vi "Final Project GUI SIM VERSION .vi"() -> ()   [LabVIEW 2021]
uses:
  <vilib>/picture/picture.llb/Draw True-Color Pixmap.vi
  <vilib>/addons/control/pid/NI_PID_pid.lvlib
  <vilib>/addons/control/pid/pid.llb/PID (DBL).vi
panel:
  out "Rear Left Actuator":string
  out "Front Left Actuator":string
  out "Rear Right Actuator":string
  out "Front Right Actuator":string
  in  "Back Button":bool
  in  "Right Button":bool
  in  "Front Button":bool
  in  "Left Button":bool
  in  "PID gains":T1={"proportional gain (Kc)"=20.0, "integral time (Ti, min)"=0.008, "derivative time (Td, min)"=0.001} {"derivative time (Td, min)" format="%.3f"; "integral time (Ti, min)" format="%.3f"; "proportional gain (Kc)" format="%.3f"}
  out "Side View":picture
  out "24-bit pixmap":u32[][](array[numeric]) format="%x"
  out "Front View":picture
  in  "Stop":bool
  # "DISTURBANCE CREATOR\n(Press a button to introduce a bump on that specific side)"
  # "CAR"
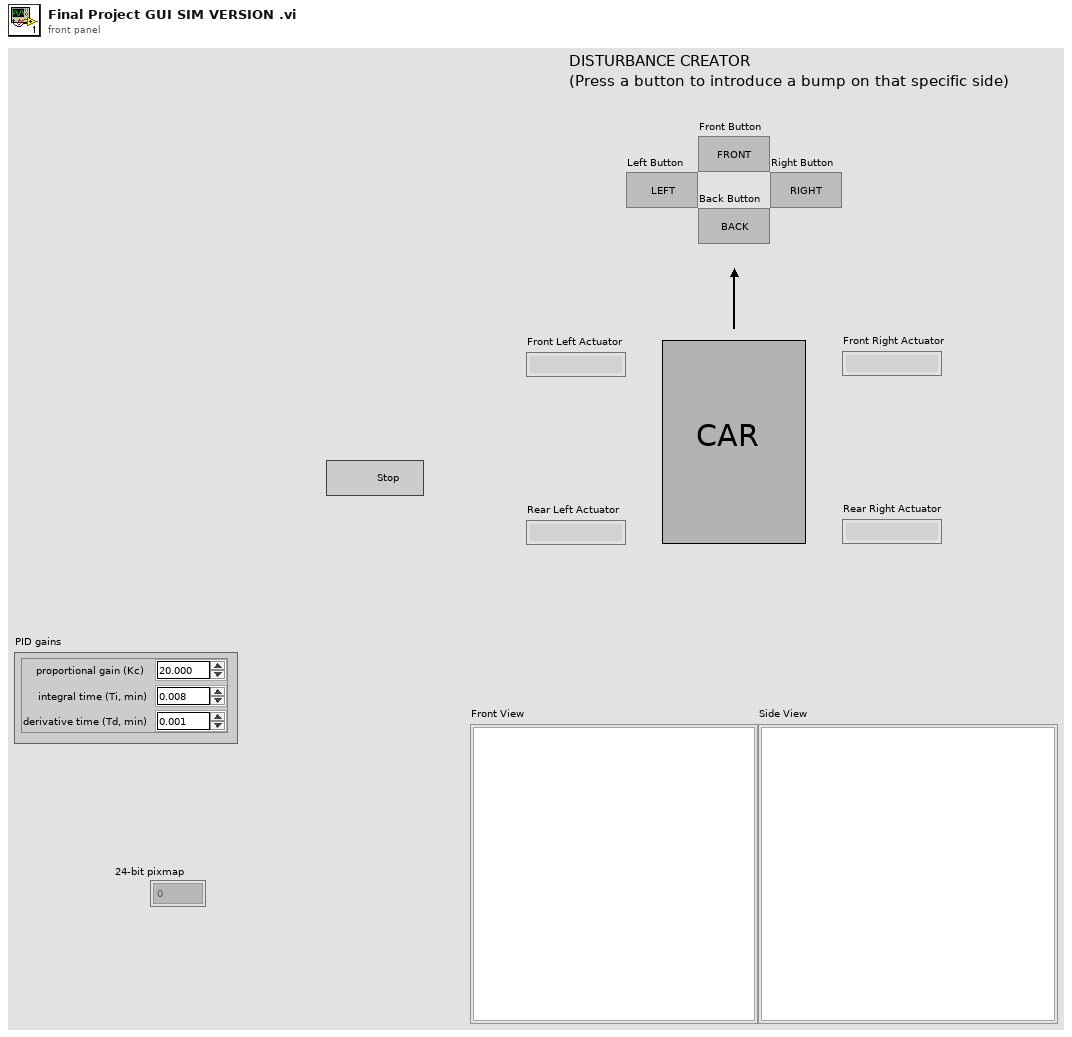
[diagram p1: front panel]
types:
  T1 = cluster{"proportional gain (Kc)":dbl, "integral time (Ti, min)":dbl, "derivative time (Td, min)":dbl}
  T2 = typedef "imagedata.ctl" = cluster{"image type":i32, "image depth":i32, "image":u8[], "mask":u8[], "colors":u32[], "Rectangle":cluster{"left":i16, "top":i16, "right":i16, "bottom":i16}}
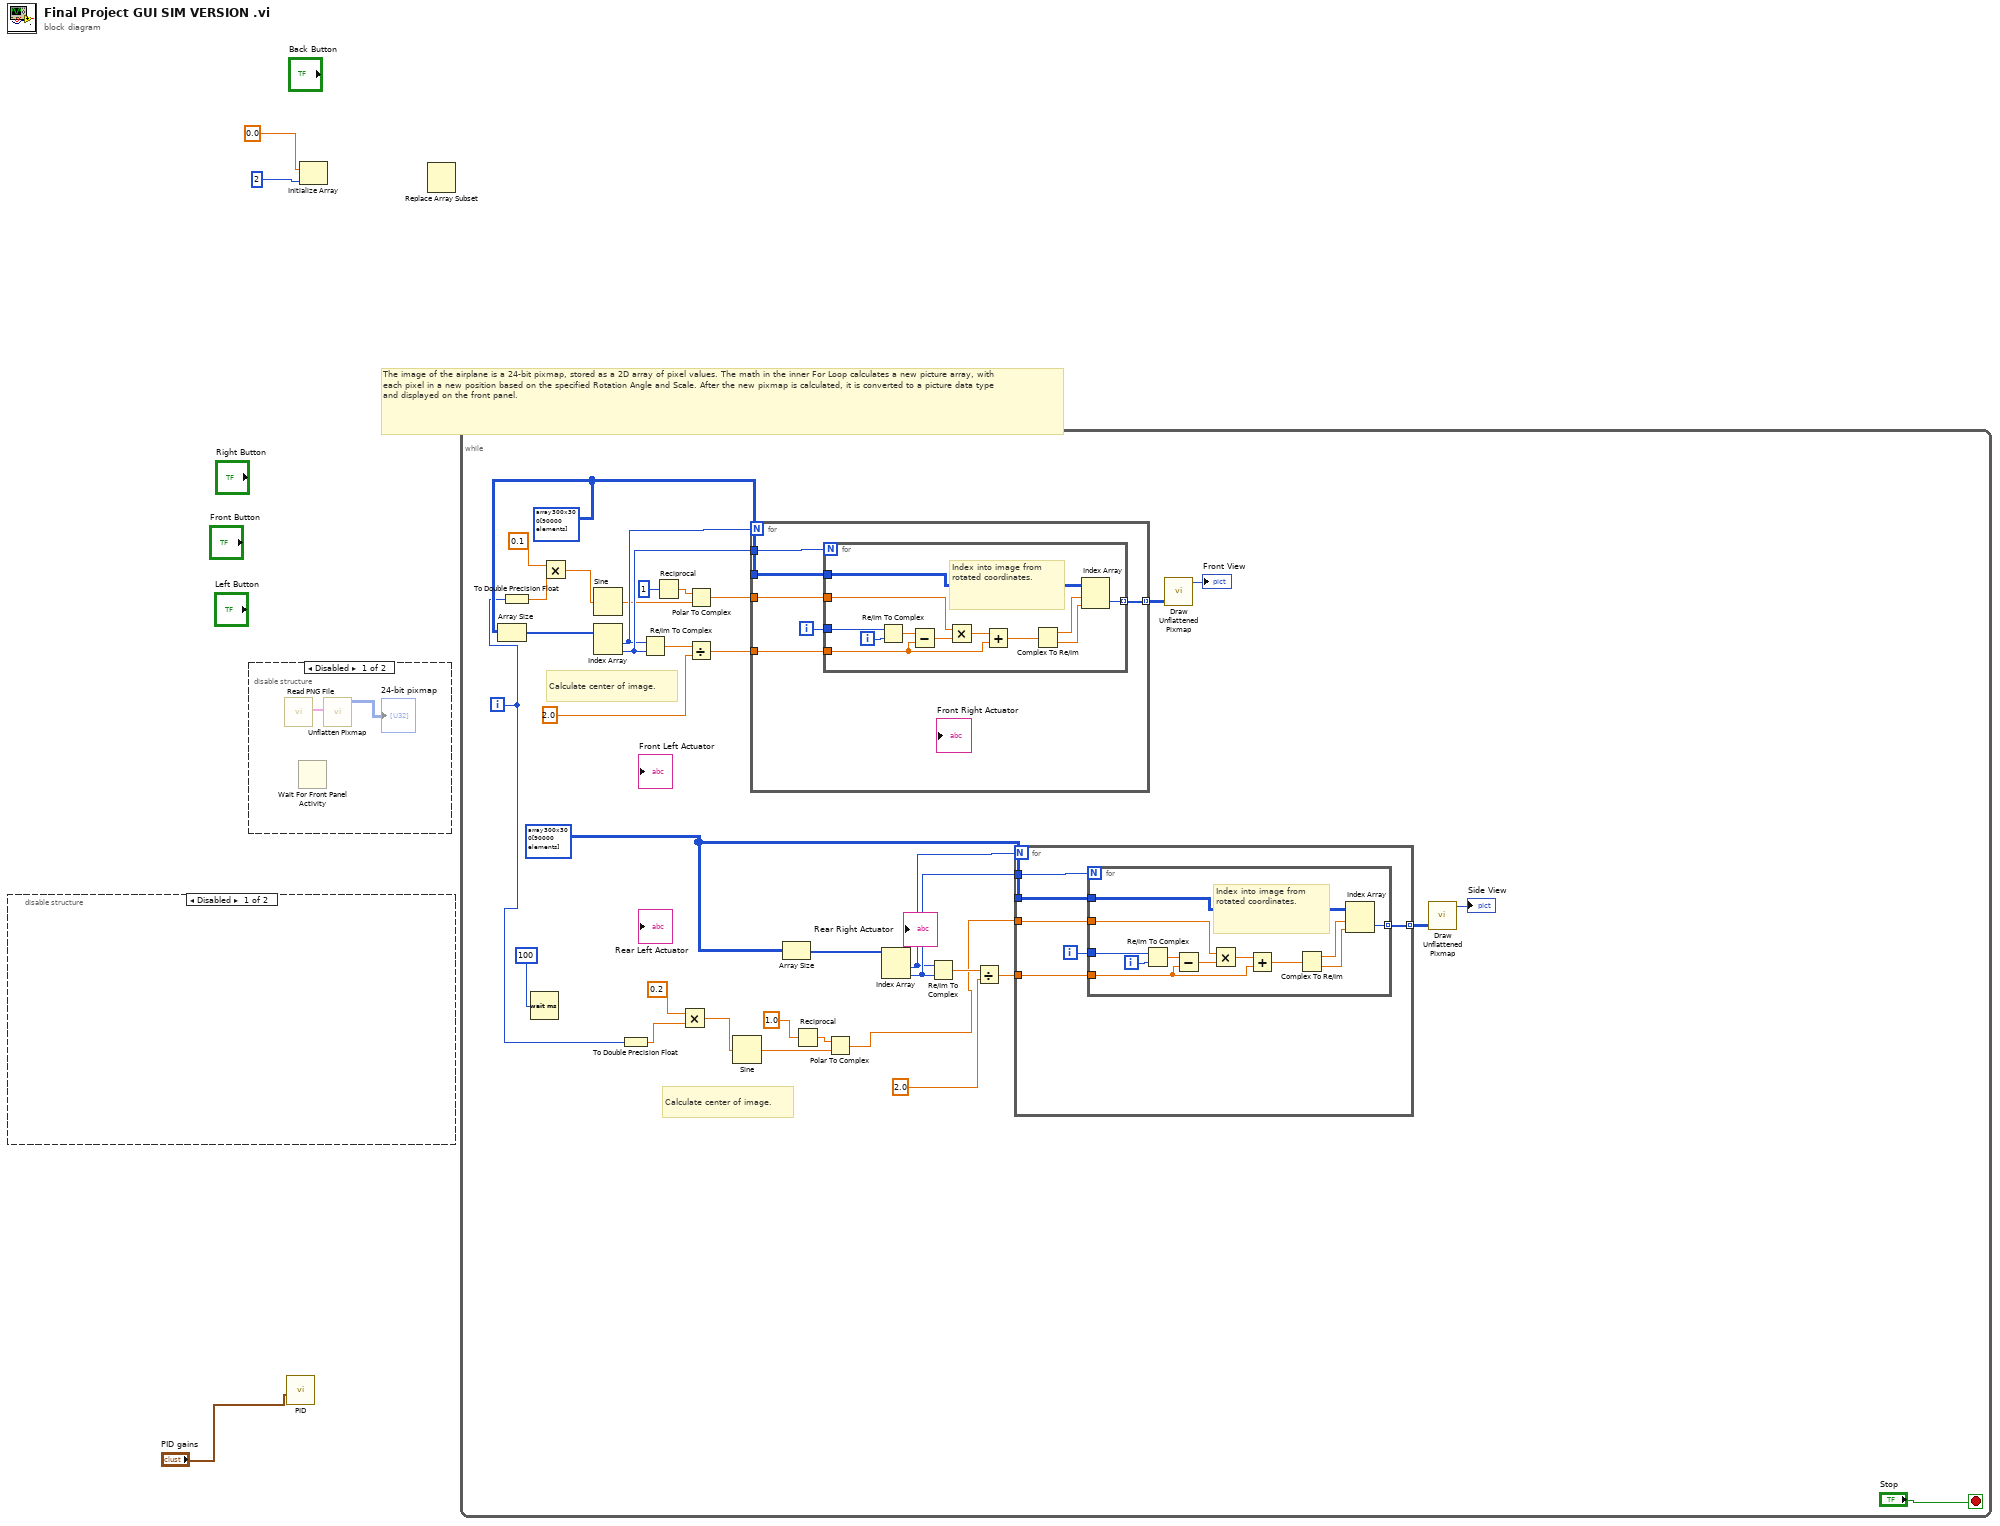
[diagram p0: block diagram]
diagram:
  # "The image of the airplane is a 24-bit pixmap, stored as a 2D array of pixel values. The math in the inner For Loop calculates a new picture array, with each pixel in a new position based on the specified Rotation Angle and Scale. After the new pixmap is calculated, it is converted to a picture data type and displayed on the front panel."
  n1 = disable-structure shown="Disabled" {
    frame Disabled {
    }
    frame Enabled {
    }
  }
  n2 = disable-structure shown="Disabled" {
    frame Disabled {
      n3 = call <vilib>:"Read PNG File.vi"() -> ("image data"=w5:T2)  [unwired: 9 in, 2 out]
      n4 = Wait For Front Panel Activity() -> ()  [unwired: 3 in, 1 out]
      n5 = call <vilib>:"Unflatten Pixmap.vi"("image data"=w5) -> ("24-bit pixmap"=→"24-bit pixmap":u32[][])  [unwired: 4 in, 6 out]
    }
    frame Enabled {
    }
  }
  n6 = call-poly <vilib>:"PID.vi"("PID gains"="PID gains") -> ()  [unwired: 9 in, 2 out]
  n7 = Initialize Array(0.0, 2) -> ()  [unwired: 1 out]
  n8 = Replace Array Subset() -> ()  [unwired: 3 in, 1 out]
  n9 = while {
    i -> [w9]
    stop <- "Stop" stop-if-true
    w11 = u32[][] array300x300[90000 elements] ("24-bit pixmap")
    w18 = u32[][] array300x300[90000 elements] ("24-bit pixmap")
    # "Calculate center of image."
    # "Calculate center of image."
    n10 = Array Size(array=w18) -> (size(s)=w36:i32[])
    n11 = To Double Precision Float(number=w9) -> (double precision float=w28:dbl)
    n12 = Wait (ms)(milliseconds to wait=u32 100) -> ()  [unwired: 1 out]
    n13 = Multiply(x=0.1, y=w28) -> (x*y=w20:dbl)
    n14 = Sine(x=w20) -> (sin(x)=w31:dbl)
    n15 = Index Array(array=w36) -> (element #1=w34:i32, element #2=w35:i32)  [unwired: 2 in]
    n16 = To Double Precision Float(number=w9) -> (double precision float=w10:dbl)
    n17 = Re/Im To Complex(1:w35, 2:w34) -> (0:w37:cdb)
    n18 = Reciprocal(x=1) -> (1/x=w38:dbl)
    n19 = Multiply(x=0.2, y=w10) -> (x*y=w13:dbl)
    n20 = Polar To Complex(1:w31, 2:w38) -> (0:w19:cdb)
    n21 = Divide(x=w37, y=2.0) -> (x/y=w33:cdb)
    n22 = Sine(x=w13) -> (sin(x)=w15:dbl)
    n23 = for {
      N: w34 -> [_]
      tunnel: w35 -> [w63]
      tunnel: w18 -> [w62]
      tunnel: [w61] -> w40 mode=indexing
      tunnel: w19 -> [w60]
      tunnel: w33 -> [w59]
      i -> [w64]
      n24 = for {
        N: w63 -> [_]
        tunnel: w64 -> [w73]
        tunnel: w62 -> [w76]
        tunnel: [w75] -> w61 mode=indexing
        tunnel: w60 -> [w70]
        tunnel: w59 -> [w65]
        i -> [w74]
        # "Index into image from rotated coordinates."
        n25 = Re/Im To Complex(1:w74, 2:w73) -> (0:w72:cdb)
        n26 = Subtract(x=w72, y=w65) -> (x-y=w71:cdb)
        n27 = Multiply(x=w70, y=w71) -> (x*y=w69:cdb)
        n28 = Add(x=w69, y=w65) -> (x+y=w68:cdb)
        n29 = Complex To Re/Im(x + iy=w68) -> (x=w67:dbl, y=w66:dbl)
        n30 = Index Array(array=w76, index (row)=w67, index (col)=w66) -> (element=w75:u32)
      }
    }
    n31 = Array Size(array=w11) -> (size(s)=w21:i32[])
    n32 = Reciprocal(x=1.0) -> (1/x=w17:dbl)
    n33 = Polar To Complex(1:w15, 2:w17) -> (0:w8:cdb)
    n34 = Index Array(array=w21) -> (element #1=w23:i32, element #2=w24:i32)  [unwired: 2 in]
    n35 = Re/Im To Complex(1:w24, 2:w23) -> (0:w25:cdb)
    n36 = Divide(x=w25, y=2.0) -> (x/y=w22:cdb)
    n37 = for {
      N: w23 -> [_]
      tunnel: w24 -> [w45]
      tunnel: w11 -> [w44]
      tunnel: [w43] -> w27 mode=indexing
      tunnel: w8 -> [w42]
      tunnel: w22 -> [w41]
      i -> [w46]
      n38 = for {
        N: w45 -> [_]
        tunnel: w46 -> [w55]
        tunnel: w44 -> [w58]
        tunnel: [w57] -> w43 mode=indexing
        tunnel: w42 -> [w52]
        tunnel: w41 -> [w47]
        i -> [w56]
        # "Index into image from rotated coordinates."
        n39 = Re/Im To Complex(1:w56, 2:w55) -> (0:w54:cdb)
        n40 = Subtract(x=w54, y=w47) -> (x-y=w53:cdb)
        n41 = Multiply(x=w52, y=w53) -> (x*y=w51:cdb)
        n42 = Add(x=w51, y=w47) -> (x+y=w50:cdb)
        n43 = Complex To Re/Im(x + iy=w50) -> (x=w49:dbl, y=w48:dbl)
        n44 = Index Array(array=w58, index (row)=w49, index (col)=w48) -> (element=w57:u32)
      }
    }
    n45 = call-poly <vilib>:"Draw Unflattened Pixmap.vi"("data (RGB format)"=w40) -> ("new picture"=→"Front View":picture)  [unwired: 8 in]
    n46 = call-poly <vilib>:"Draw Unflattened Pixmap.vi"("data (RGB format)"=w27) -> ("new picture"=→"Side View":picture)  [unwired: 8 in]
  }
